vi "Configure Gate Time.vi"(0 "VISA resource name":refnum<visa-resource-name>, 1 "Enable Gate (F: Disable)":bool, 2 "Gate Length (0.0004616 s)":dbl=0.0004616, 5 "Gate Delay (5.77E-5 s)":dbl=5.77e-05, 7 "Gate Method (0: LO)":i32(ring) items=["LO", "Video", "FFT"], 9 "Gate Source (0: Line)":i32(ring) items=["Line", "External1", "External2", "RF Burst", "Periodic Timer"], 11 "error in (no error)":errorcluster, 12 "Gate Control (0: Edge)":i32(ring) items=["Edge", "Level"]) -> (4 "VISA resource name out":refnum<visa-resource-name>, 15 "error out":errorcluster)   [LabVIEW 2018, in "Agilent MXA Series.lvlib"]
doc: "Configures the gating function."
uses:
  Agilent MXA Series.lvlib
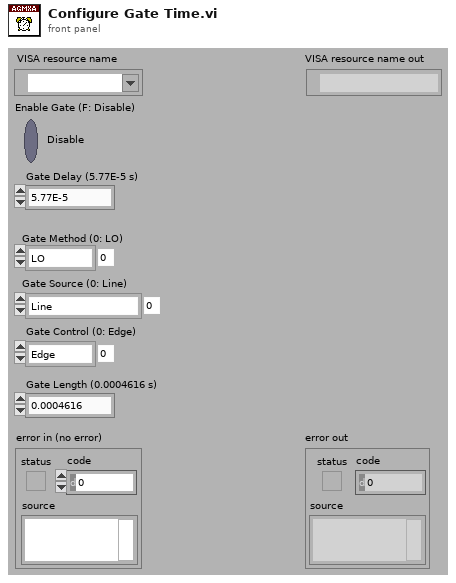
[diagram p1: front panel]
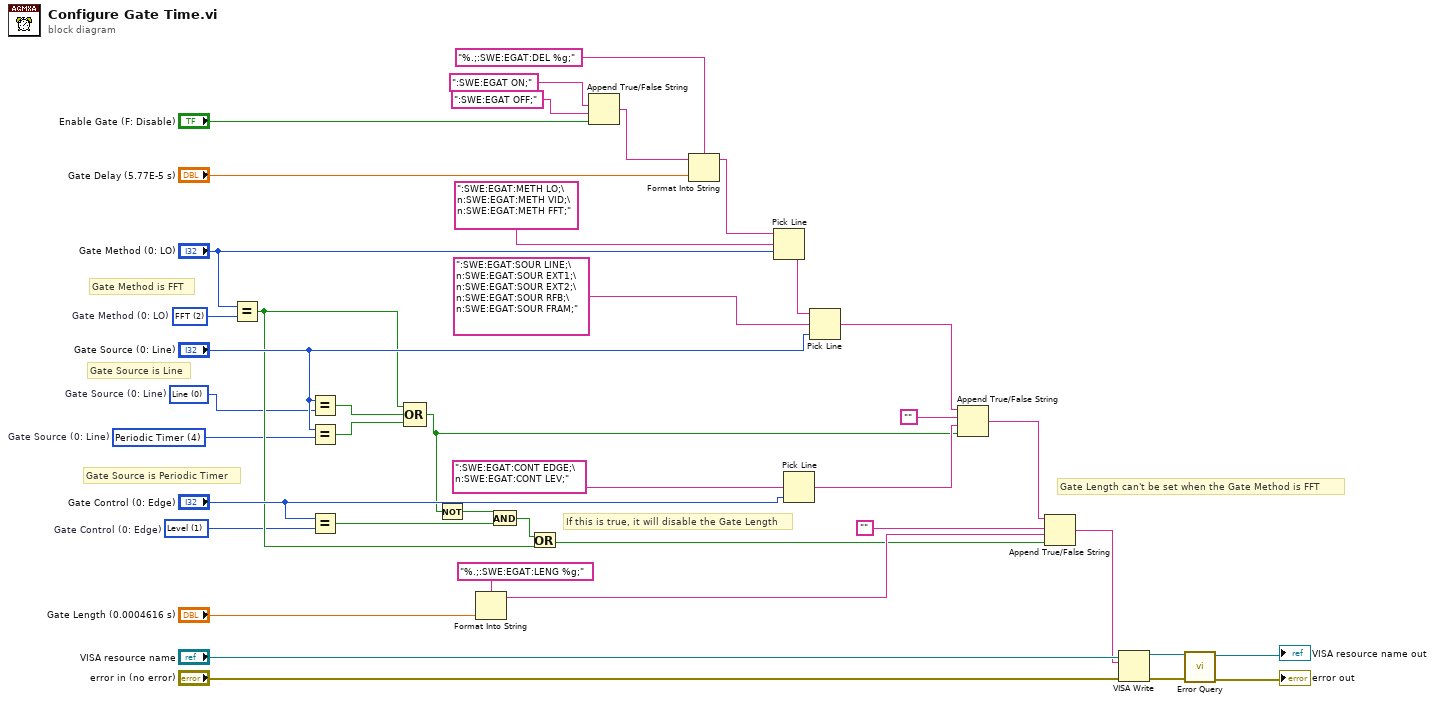
[diagram p0: block diagram]
diagram:
  w1 = 4 items=["Line", "External1", "External2", "RF Burst", "Periodic Timer"]  # Gate Source (0: Line)
  w2 = 1 items=["Edge", "Level"]  # Gate Control (0: Edge)
  w3 = 0 items=["Line", "External1", "External2", "RF Burst", "Periodic Timer"]  # Gate Source (0: Line)
  w4 = 2 items=["LO", "Video", "FFT"]  # Gate Method (0: LO)
  # "If this is true, it will disable the Gate Length"
  # "Gate Length can't be set when the Gate Method is FFT"
  # "Gate Method is FFT"
  # "Gate Source is Periodic Timer"
  # "Gate Source is Line"
  n1 = Equal?(x="Gate Method (0: LO)", y=w4) -> (x = y?=w7:bool)
  n2 = Equal?(x="Gate Source (0: Line)", y=w3) -> (x = y?=w26:bool)
  n3 = Equal?(x="Gate Source (0: Line)", y=w1) -> (x = y?=w25:bool)
  n4 = Equal?(x="Gate Control (0: Edge)", y=w2) -> (x = y?=w15:bool)
  n5 = Compound Arithmetic op=OR(w7, w26, w25) -> (w14:bool)
  n6 = Not(x=w14) -> (.not. x?=w13:bool)
  n7 = Format Into String(format string="%.;:SWE:EGAT:LENG %g;", "Gate Length (0.0004616 s)") -> (resulting string=w20:string)  [unwired: 2 in, 1 out]
  n8 = And(x=w13, y=w15) -> (x .and. y?=w5:bool)
  n9 = Or(x=w5, y=w7) -> (x .or. y?=w6:bool)
  n10 = Append True/False String(1:"Enable Gate (F: Disable)", 2:":SWE:EGAT OFF;" ("false string"), 3:":SWE:EGAT ON;" ("true string")) -> (0:w27:string)  [unwired: 1 in]
  n11 = Format Into String(format string="%.;:SWE:EGAT:DEL %g;", initial string=w27, "Gate Delay (5.77E-5 s)") -> (resulting string=w12:string)  [unwired: 1 in, 1 out]
  n12 = Pick Line(string ("")=w12, multi-line string=":SWE:EGAT:METH LO;\n:SWE:EGAT:METH VID;\n:SWE:EGAT:METH FFT;", line index="Gate Method (0: LO)") -> (output string=w11:string)
  n13 = Pick Line(multi-line string=":SWE:EGAT:CONT EDGE;\n:SWE:EGAT:CONT LEV;", line index="Gate Control (0: Edge)") -> (output string=w24:string)  [unwired: 1 in]
  n14 = Pick Line(string ("")=w11, multi-line string=":SWE:EGAT:SOUR LINE;\n:SWE:EGAT:SOUR EXT1;\n:SWE:EGAT:SOUR EXT2;\n:SWE:EGAT:SOUR RFB;\n:SWE:EGAT:SOUR FRAM;", line index="Gate Source (0: Line)") -> (output string=w10:string)
  n15 = Append True/False String(1:w14, 2:w24, 3:"" ("true string"), 4:w10) -> (0:w9:string)
  n16 = Append True/False String(1:w6, 2:w20, 3:"", 4:w9) -> (0:w8:string)
  n17 = VISA Write(VISA resource name="VISA resource name", write buffer=w8, error in (no error)="error in (no error)") -> (VISA resource name out=w31:refnum<visa-resource-name>, error out=w32:errorcluster)  [unwired: 1 out]
  n18 = call "Error Query.vi"("error in (no error)"=w32, "VISA resource name"=w31) -> ("error out"=→"error out":errorcluster, "VISA resource name out"=→"VISA resource name out":refnum<visa-resource-name>)  [unwired: 6 in, 2 out]
